vi "CreateDAQmxTaskFromP2P.vi"(0 "DAQmx Device Name":tag) -> (1 "task out":refnum<k21>, 2 "Extra Properties":string[][](array[string]))   [LabVIEW 2018]
uses:
  Global Variables.vi
  <vilib>/DAQmx/create/channels.llb/DAQmx Create Channel (AI-Current-Basic).vi
  <vilib>/DAQmx/create/channels.llb/DAQmx Create Channel (AI-Voltage-Basic).vi
  <vilib>/DAQmx/create/channels.llb/DAQmx Create Channel (AI-Temperature-Thermocouple).vi
  <resource>/objmgr/daqmx.rc
panel:
  in  "AI.Thrmcpl.Type":i32(ring)=10072 items=["J"=10072, "K"=10073, "N"=10077, "R"=10082, "S"=10085, "T"=10086, "B"=10047, "E"=10055]
  out "AI.MeasTypes":i32[](array[ring]) items=["Voltage"=10322, "Voltage RMS"=10350, "Current"=10134, "Current RMS"=10351, "More:Voltage:Custom with Excitation"=10323, "More:Bridge (V/V)"=15908, "Frequency"=10181, "Resistance"=10278, "Temperature:Thermocouple"=10303, "Temperature:Thermistor"=10302, "Temperature:RTD"=10301, "Temperature:Built-in Sensor"=10311, "Strain Gage"=10300, "Rosette Strain Gage"=15980, "Position:LVDT"=10352, "Position:RVDT"=10353, "Position:Eddy Current Proximity Probe"=14835, "Accelerometer"=10356, "Acceleration:Charge"=16104, "Acceleration:4 Wire DC Voltage"=16106, "Velocity:IEPE Sensor"=15966, "Force:Bridge"=15899, "Force:IEPE Sensor"=15895, "Pressure:Bridge"=15902, "Sound Pressure:Microphone"=10354, "Torque:Bridge"=15905, "TEDS Sensor"=12531, "Charge"=16105]
  out "Channels":refnum<k21>[](array[refnum])
  out "Input Type":string
  out "Array In":string[][](array[string])
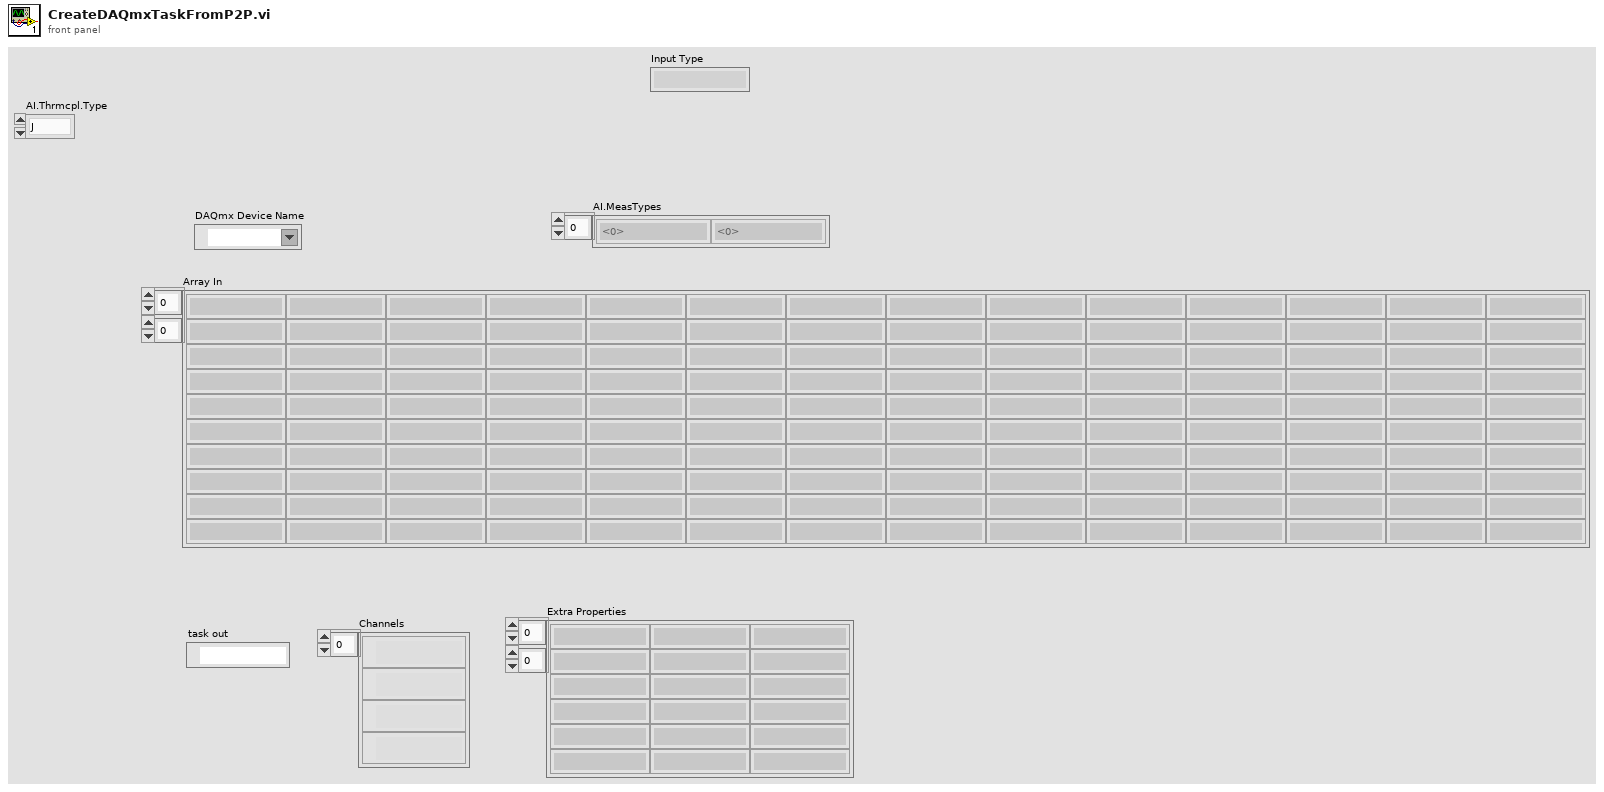
[diagram p1: front panel]
types:
  T1 = typedef "LVStringsAndValuesArrayTypeDef_I32.ctl" = cluster{"String":string, "Value":i32}[]
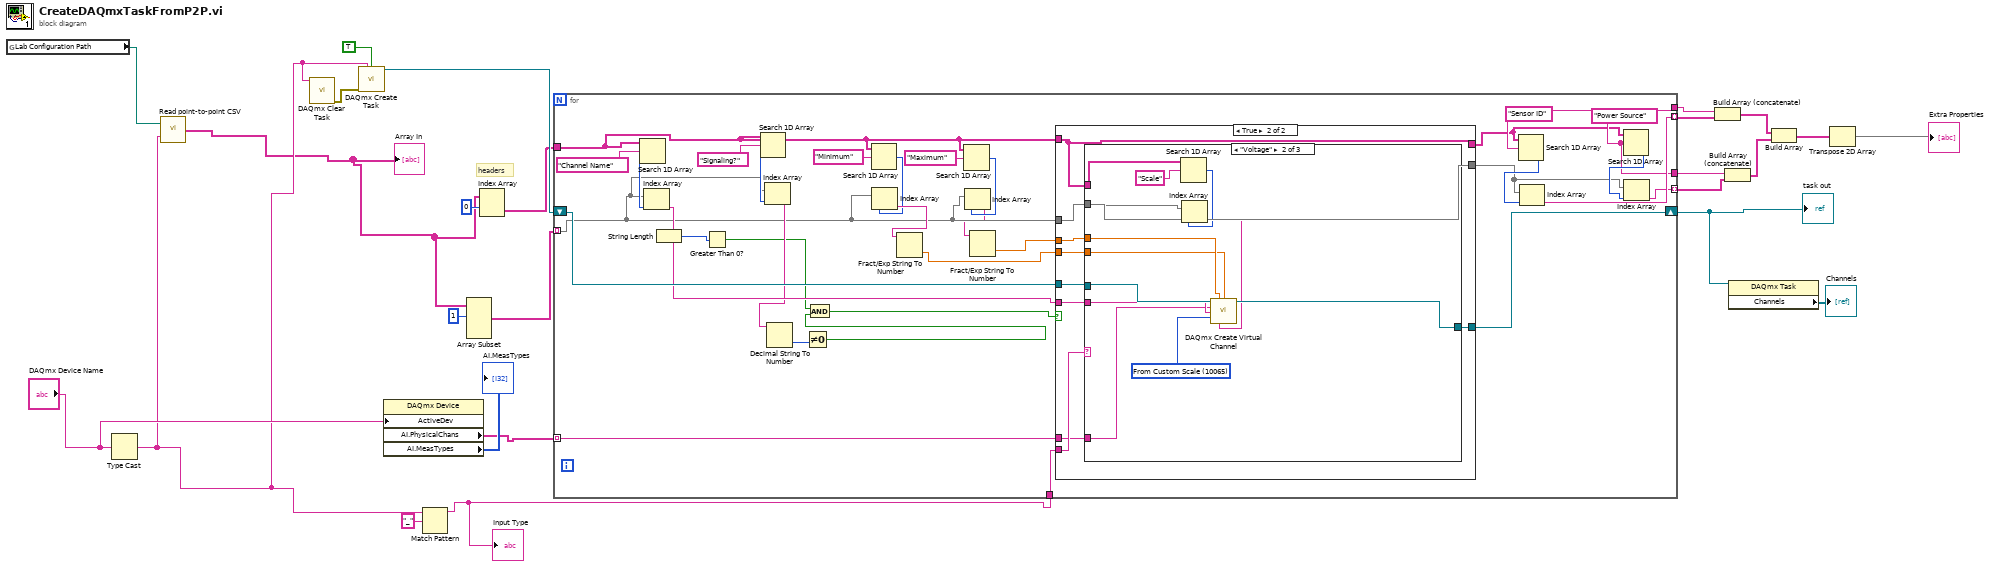
[diagram p0: block diagram]
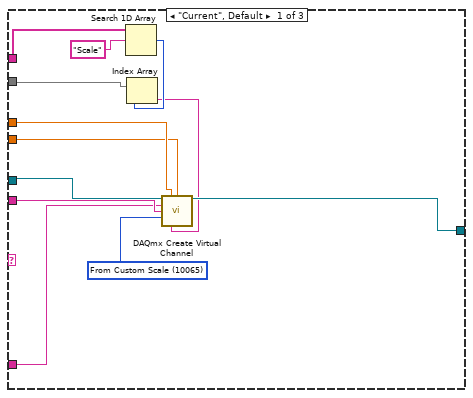
[diagram p3: hidden frame]
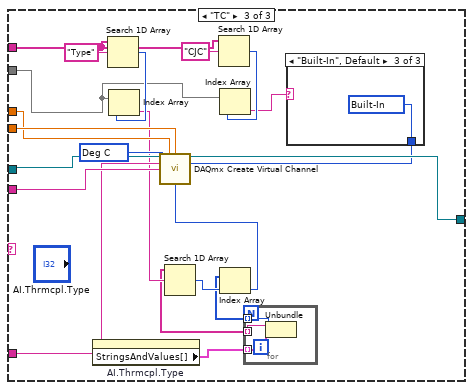
[diagram p4: hidden frame]
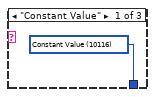
[diagram p5: hidden frame]
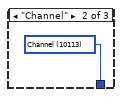
[diagram p6: hidden frame]
diagram:
  # "headers"
  n1 = global read "Global Variables.vi" "Lab Configuration Path"() -> (w1:path)
  n2 = Type Cast(x="DAQmx Device Name") -> (*(type *) &x=w3:string)  [unwired: 1 in]
  n3 = call "Read point-to-point CSV.vi"("Device Name"=w3, "Path"=w1) -> ("Array Out"=w2:string[][])
  "Array In" <- w2
  n4 = call <vilib>:"DAQmx Clear Task.vi"("task in"=w3) -> ("error out"=w23:errorcluster)  [unwired: 14 in]
  n5 = call <vilib>:"DAQmx Create Task.vi"("new task name"=w3, "auto cleanup"=TRUE, "error in"=w23) -> ("task out"=w25:refnum<k21>)  [unwired: 11 in, 1 out]
  n6 = property class="DAQmx Device"("ActiveDev"="DAQmx Device Name") -> ("AI.PhysicalChans"=w4:tag[], "AI.MeasTypes"=→"AI.MeasTypes":i32[])  [unwired: 2 in, 2 out]
  n7 = Match Pattern(string=w3, regular expression="_") -> (before substring=w10:string)  [unwired: 1 in, 3 out]
  "Input Type" <- w10
  n8 = Array Subset(array=w2, index (row)=1 ("index")) -> (w21:string[][])  [unwired: 3 in]
  n9 = Index Array(array=w2, index (row)=0) -> (element=w9:string[])  [unwired: 1 in]
  n10 = for {
    tunnel: w21 -> [w27] mode=indexing
    shift-right: [w57] -> w8
    shift-left: w25 -> [w58]
    tunnel: w9 -> [w28]
    tunnel: [w51] -> w18 mode=indexing
    tunnel: [w50] -> w19
    tunnel: [w48] -> w16 mode=indexing
    tunnel: [w47] -> w17
    tunnel: w10 -> [w46]
    tunnel: w4 -> [w43] mode=indexing
    w47 = "Power Source" ("element")
    w50 = "Sensor ID" ("element")
    n11 = Search 1D Array(1D array=w28, element="Channel Name") -> (index of element=w53:i32)  [unwired: 1 in]
    n12 = Index Array(array=w27, index=w53) -> (element=w55:string)
    n13 = String Length(string=w55) -> (length=w56:i32)
    n14 = Greater Than 0?(x=w56) -> (x > 0?=w37:bool)
    n15 = Search 1D Array(1D array=w28, element="Signaling?") -> (index of element=w42:i32)  [unwired: 1 in]
    n16 = Index Array(array=w27, index=w42) -> (element=w40:string)
    n17 = Decimal String To Number(string=w40) -> (number=w39:i32)  [unwired: 2 in, 1 out]
    n18 = Not Equal To 0?(x=w39) -> (x != 0?=w38:bool)
    n19 = And(x=w37, y=w38) -> (x .and. y?=w36:bool)
    n20 = Search 1D Array(1D array=w28, element="Minimum") -> (index of element=w33:i32)  [unwired: 1 in]
    n21 = Index Array(array=w27, index=w33) -> (element=w35:string)
    n22 = Fract/Exp String To Number(string=w35) -> (number=w29:dbl)  [unwired: 3 in, 1 out]
    n23 = Search 1D Array(1D array=w28, element="Maximum") -> (index of element=w34:i32)  [unwired: 1 in]
    n24 = Index Array(array=w27, index=w34) -> (element=w26:string)
    n25 = Fract/Exp String To Number(string=w26) -> (number=w30:dbl)  [unwired: 3 in, 1 out]
    n26 = case shown="True" w36 {
      tunnel: w58 -> [w61 w70]
      tunnel: [w61 w69] -> w57
      tunnel: w55 -> [_ w68]
      tunnel: w46 -> [_ w67]
      tunnel: w27 -> [w59 w65]
      tunnel: w28 -> [w60 w66]
      tunnel: [w60 w66] -> w45
      tunnel: [w59 w65] -> w44
      tunnel: w43 -> [_ w64]
      tunnel: w30 -> [_ w63]
      tunnel: w29 -> [_ w62]
      frame False {
      }
      frame True {
        n27 = case shown="\"Voltage\"" w67 {
          tunnel: w70 -> [w82 w94 w115]
          tunnel: [w81 w93 w114] -> w69
          tunnel: w68 -> [w80 w92 w113]
          tunnel: w65 -> [w71 w83 w105]
          tunnel: w66 -> [w74 w86 w106]
          tunnel: w64 -> [w75 w87 w109]
          tunnel: w63 -> [w73 w85 w101]
          tunnel: w62 -> [w72 w84 w102]
          frame "Current", Default {
            w79 = 10065 items=["Amps"=10342, "From Custom Scale"=10065] ("units")
            n28 = Search 1D Array(1D array=w74, element="Scale") -> (index of element=w77:i32)  [unwired: 1 in]
            n29 = Index Array(array=w71, index=w77) -> (element=w76:string)
            n30 = call-poly <vilib>:"DAQmx Create Virtual Channel.vi"("task in"=w82, "maximum value"=w73, "minimum value"=w72, "physical channels"=w75, "name to assign"=w80, "units"=w79, "custom scale name"=w76) -> ("task out"=w81:refnum<k21>)  [unwired: 7 in, 1 out]
          }
          frame "Voltage" {
            w91 = 10065 items=["Amps"=10342, "From Custom Scale"=10065] ("units")
            n31 = Search 1D Array(1D array=w86, element="Scale") -> (index of element=w89:i32)  [unwired: 1 in]
            n32 = Index Array(array=w83, index=w89) -> (element=w88:string)
            n33 = call-poly <vilib>:"DAQmx Create Virtual Channel.vi"("task in"=w94, "maximum value"=w85, "minimum value"=w84, "physical channels"=w87, "name to assign"=w92, "units"=w91, "custom scale name"=w88) -> ("task out"=w93:refnum<k21>)  [unwired: 7 in, 1 out]
          }
          frame "TC" {
            w110 = 10143 items=["Deg C"=10143, "Deg F"=10144, "Kelvins"=10325, "Deg R"=10145, "From Custom Scale"=10065] ("units")
            n34 = property on="AI.Thrmcpl.Type" class="Ring (strict)"() -> ("StringsAndValues[]"=w99:T1)  [unwired: 2 in, 2 out]
            n35 = Search 1D Array(1D array=w106, element="Type") -> (index of element=w111:i32)  [unwired: 1 in]
            n36 = Index Array(array=w105, index=w111) -> (element=w100:string)
            n37 = Search 1D Array(1D array=w106, element="CJC") -> (index of element=w108:i32)  [unwired: 1 in]
            n38 = Index Array(array=w105, index=w108) -> (element=w104:string)
            n39 = for {
              tunnel: w99 -> [w118] mode=indexing
              tunnel: [w117] -> w98 mode=indexing
              tunnel: [w116] -> w96 mode=indexing
              n40 = Unbundle(w118) -> ("String"=w117:string, "Value"=w116:i32)
            }
            n41 = Search 1D Array(1D array=w98, element=w100) -> (index of element=w97:i32)  [unwired: 1 in]
            n42 = Index Array(array=w96, index=w97) -> (element=w95:i32)
            n43 = case shown="\"Built-In\", Default" w104 {
              tunnel: [w119 w120 w121] -> w103
              frame "Constant Value" {
                w119 = 10116 items=["Built-In"=10200, "Constant Value"=10116, "Channel"=10113] ("cjc source")
              }
              frame "Channel" {
                w120 = 10113 items=["Built-In"=10200, "Constant Value"=10116, "Channel"=10113] ("cjc source")
              }
              frame "Built-In", Default {
                w121 = 10200 items=["Built-In"=10200, "Constant Value"=10116, "Channel"=10113] ("cjc source")
              }
            }
            n44 = call-poly <vilib>:"DAQmx Create Virtual Channel.vi"("task in"=w115, "maximum value"=w101, "minimum value"=w102, "physical channels"=w109, "cjc source"=w103, "name to assign"=w113, "units"=w110, "thermocouple type"=w95) -> ("task out"=w114:refnum<k21>)  [unwired: 6 in, 1 out]
          }
        }
      }
    }
    n45 = Search 1D Array(1D array=w45, element=w50) -> (index of element=w52:i32)  [unwired: 1 in]
    n46 = Index Array(array=w44, index=w52) -> (element=w51:string)
    n47 = Search 1D Array(1D array=w45, element=w47) -> (index of element=w49:i32)  [unwired: 1 in]
    n48 = Index Array(array=w44, index=w49) -> (element=w48:string)
  }
  "task out" <- w8
  n49 = Build Array (concatenate)(w19, w18) -> (w15:string[])
  n50 = Build Array (concatenate)(w17, w16) -> (w14:string[])
  n51 = property class="DAQmx Task"(reference=w8) -> ("Channels"=→"Channels":refnum<k21>[])  [unwired: 1 in, 2 out]
  n52 = Build Array(w15, w14) -> (w13:string[][])
  n53 = Transpose 2D Array(2D array=w13) -> (transposed array=→"Extra Properties":string[][])
